vi "Execute.vi"(8 "error in (no error)":errorcluster, 10 "System In":refnum<class "abs_System.lvclass">, 11 "Node in":refnum<class "Test Boolean.lvclass">) -> (0 "error out":errorcluster, 1 "Status":T1, 2 "System Out":refnum<class "abs_System.lvclass">, 3 "Node out":refnum<class "Test Boolean.lvclass">)   [LabVIEW 2021, in "Test Boolean.lvclass"]
uses:
  Test Boolean.lvclass
  C:/Users/Tim/Documents/GitHub/LV_Behaviour_Tree/Source/Support/abs_Type Leaf/abs_Type Leaf.lvclass
  abs_Node/Status.ctl
  abs_System/abs_System.lvclass
  LV_Abstract/Source/Abs_Types/Boolean/Abs_Boolean.lvclass
  C:/Users/Tim/Documents/GitHub/LV_Abstract/Source/Abs_Types/Type/Abs_Type.lvclass
  abs_Type Leaf/abs_Type Leaf.lvclass/abs_Type Leaf.ctl
  abs_Type Leaf/Properties/Read Value Class.vi
  abs_Type Leaf/Properties/Write Value Class.vi
  LV_Abstract/Source/Abs_Types/Type/Abs_Type.lvclass
  abs_Type Leaf/abs_Type Leaf.lvclass
  abs_Node/abs_Node.lvclass
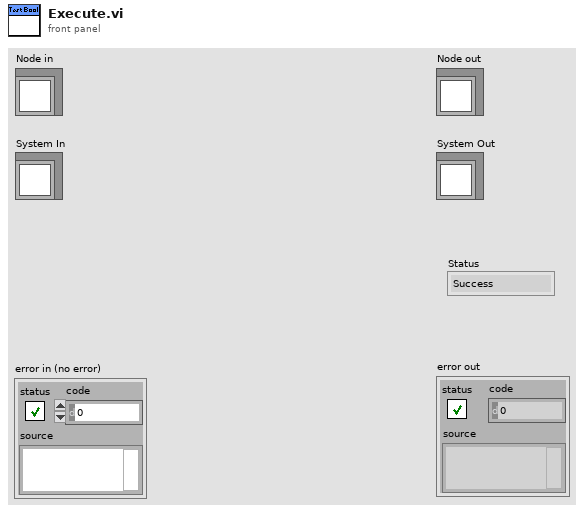
[diagram p1: front panel]
types:
  T1 = typedef "BT.lvlib/abs_Node.lvclass/Status.ctl" = enum16{"Success", "Failure", "Running"}
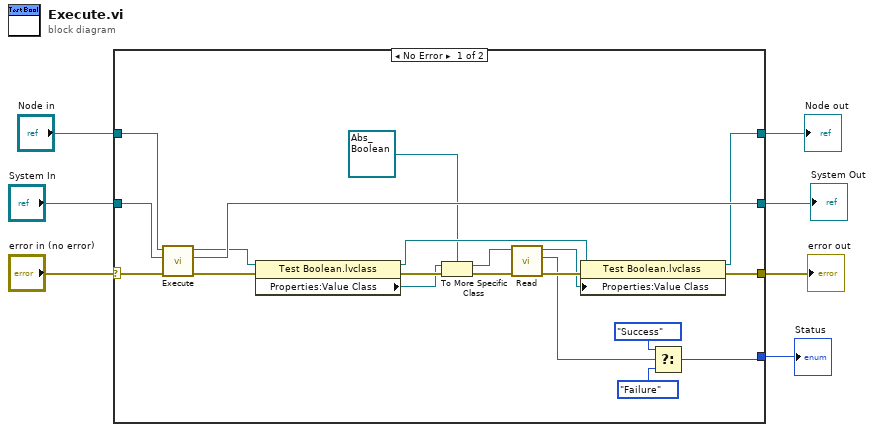
[diagram p0: block diagram]
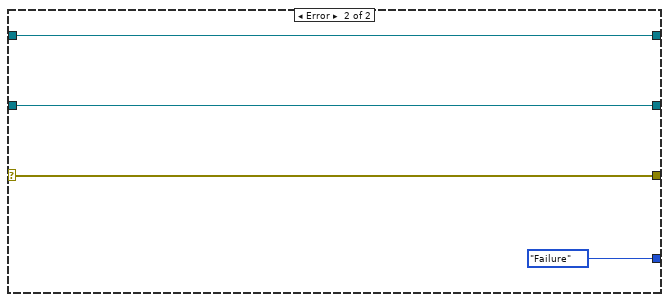
[diagram p2: hidden frame]
diagram:
  n1 = case shown="No Error" "error in (no error)" {
    selector: "error in (no error)" -> [w26 w29]
    tunnel: [w27 w30] -> w3
    tunnel: "System In" -> [w25 w30]
    tunnel: "Node in" -> [w24 w31]
    tunnel: [w20 w29] -> w4
    tunnel: [w19 w31] -> w2
    tunnel: [w18 Status."Failure" ("Status")] -> w1
    frame No Error {
      n2 = call-parent "Execute.vi"("error in (no error)"=w26, "System In"=w25, "Node in"=w24) -> ("error out"=w23:errorcluster, "System Out"=w27:refnum<class "abs_System.lvclass">, "Node out"=w22:refnum<class "Test Boolean.lvclass">)  [unwired: 5 in, 1 out]
      n3 = property class="Test Boolean.lvclass"(reference=w22, error in=w23) -> (reference out=w21:refnum<class "Test Boolean.lvclass">, error out=w14:errorcluster, "Properties:Value Class"=w12:refnum<class "Abs_Type.lvclass">)
      n4 = To More Specific Class(target class=refnum<class "Abs_Boolean.lvclass"> refnum ("Boolean in"), reference=w12, error in=w14) -> (specific class reference=w10:refnum<class "Abs_Boolean.lvclass">, error out=w13:errorcluster)
      n5 = call-dynamic "Read.vi"("error in (no error)"=w13, "Boolean in"=w10) -> ("error out"=w17:errorcluster, "Boolean"=w15:bool, "Boolean out"=w16:refnum<class "Abs_Boolean.lvclass">)  [unwired: 7 in]
      n6 = property class="Test Boolean.lvclass"(reference=w21, error in=w17, "Properties:Value Class"=w16) -> (reference out=w19:refnum<class "Test Boolean.lvclass">, error out=w20:errorcluster)
      n7 = Select(t=Status."Success" ("Status"), s=w15, f=Status."Failure" ("Status")) -> (s? t:f=w18:T1)
    }
    frame Error {
    }
  }
  "error out" <- w4
  "Node out" <- w2
  "Status" <- w1
  "System Out" <- w3
